vi "Calculate Tau Error.vi"(0 "CalErr?":bool, 1 "tau":dbl, 2 "Dt":dbl, 3 "X":dbl[](array[numeric]), 4 "A":dbl, 8 "B":dbl) -> (7 "e_tau":dbl)   [LabVIEW 2011]
doc: "Calculate the error in the fitted coefficient tau according to Halmer et al. [2004, Rev. Sci. Instr.]. The error will be the standard deviation of the fit (with N-3 degrees of freedom) multiplied by the sum of the square of the derivative of the exponential equation at each point in time."
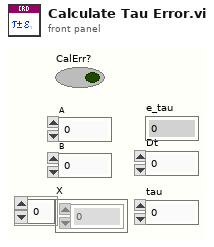
[diagram p1: front panel]
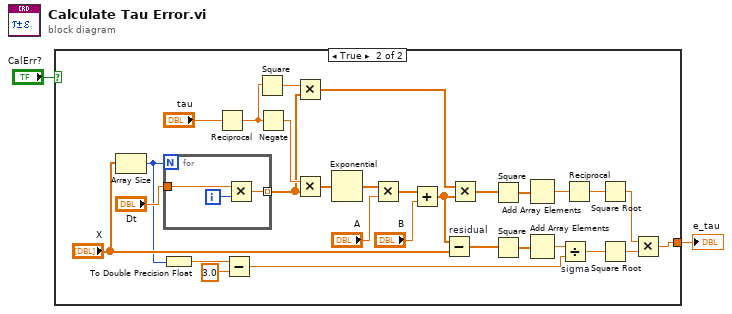
[diagram p0: block diagram]
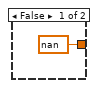
[diagram p2: hidden frame]
diagram:
  n1 = case shown="True" "CalErr?" {
    tunnel: [nan w15] -> w1
    frame False {
    }
    frame True {
      n2 = Array Size(array="X") -> (size(s)=w14:i32)
      n3 = for {
        N: w14 -> [_]
        tunnel: "Dt" -> [w34]
        tunnel: [w33] -> w20 mode=indexing
        i -> [w35]
        n4 = Multiply(x=w34, y=w35) -> (x*y=w33:dbl)
      }
      n5 = To Double Precision Float(number=w14) -> (double precision float=w31:dbl)
      n6 = Reciprocal(x="tau") -> (1/x=w22:dbl)
      n7 = Subtract(x=w31, y=3.0) -> (x-y=w30:dbl)
      n8 = Square(x=w22) -> (x^2=w21:dbl)
      n9 = Negate(x=w22) -> (-x=w25:dbl)
      n10 = Multiply(x=w21, y=w20) -> (x*y=w19:dbl[])
      n11 = Multiply(x=w25, y=w20) -> (x*y=w26:dbl[])
      n12 = Exponential(1:w26) -> (0:w8:dbl[])
      n13 = Multiply(x=w8, y="A") -> (x*y=w6:dbl[])
      n14 = Add(x=w6, y="B") -> (x+y=w4:dbl[])
      n15 = Subtract "residual"(x=w4, y="X") -> (x-y=w13:dbl[])
      n16 = Multiply(x=w19, y=w4) -> (x*y=w18:dbl[])
      n17 = Square(x=w18) -> (x^2=w17:dbl[])
      n18 = Square(x=w13) -> (x^2=w27:dbl[])
      n19 = Add Array Elements(numeric array=w17) -> (sum=w10:dbl)
      n20 = Add Array Elements(numeric array=w27) -> (sum=w28:dbl)
      n21 = Divide "sigma"(x=w28, y=w30) -> (x/y=w12:dbl)
      n22 = Reciprocal(x=w10) -> (1/x=w9:dbl)
      n23 = Square Root(x=w9) -> (sqrt(x)=w16:dbl)
      n24 = Square Root(x=w12) -> (sqrt(x)=w11:dbl)
      n25 = Multiply(x=w16, y=w11) -> (x*y=w15:dbl)
    }
  }
  "e_tau" <- w1
